vi "v4.11.vi"() -> ()   [LabVIEW 2018]
uses:
  <vilib>/DAQmx/read.llb/DAQmx Read (Analog 1D DBL NChan 1Samp).vi
  <extravilib>/ChannelInstances/High Speed Stream-c(a[.](c(dbl,dbl,dbl,dbl)),stamp,a[.](dbl),c(dbl,dbl,dbl,dbl,dbl,dbl,dbl))/_Read For Replicate.vi
  <extravilib>/ChannelInstances/High Speed Stream-c(a[.](c(dbl,dbl,dbl,dbl)),stamp,a[.](dbl),c(dbl,dbl,dbl,dbl,dbl,dbl,dbl))/Instantiate.vi
  <extravilib>/ChannelInstances/High Speed Stream-c(a[.](c(dbl,dbl,dbl,dbl)),stamp,a[.](dbl),c(dbl,dbl,dbl,dbl,dbl,dbl,dbl))/)Channel.vi
  <extravilib>/ChannelInstances/High Speed Stream-c(a[.](c(dbl,dbl,dbl,dbl)),stamp,a[.](dbl),c(dbl,dbl,dbl,dbl,dbl,dbl,dbl))/Abort Signal/Init Signal.vi
  <vilib>/Utility/file.llb/Write Delimited Spreadsheet (string).vi
  <vilib>/DAQmx/create/channels.llb/DAQmx Create Channel (AI-Temperature-Thermocouple).vi
  <vilib>/DAQmx/configure/timing.llb/DAQmx Timing (Sample Clock).vi
  <vilib>/DAQmx/miscellaneous.llb/DAQmx Fill In Error Info.vi
  <extravilib>/ChannelInstances/High Speed Stream-c(a[.](c(dbl,dbl,dbl,dbl)),stamp,a[.](dbl),c(dbl,dbl,dbl,dbl,dbl,dbl,dbl)).lvlib
  <resource>/objmgr/daqmx.rc
panel:
  out "Current Time":timestamp format="%<%X\n%x>T"
  out "Actual Sample Rate":dbl
  out "Rig Temperatures":T1
  out "Flowrate Data":T2(array[cluster])
  out "UI Timestamp":timestamp format="%<%X\n%x>T"
  out "DAQ Timestamp":timestamp format="%<%H:%M:%S>T"
  in  "file path (dialog if empty)":path
  out "Output\nStatus":T3(ring)
  in  "Start Recording?":bool
  in  "Stop Recording?":bool
  in  "Flowrate Control":dbl
  out "Status":T4(ring)
  in  "OK Button":bool
  in  "DAQ Properties":cluster{"Sample Rate [Hz]":dbl}={"Sample Rate [Hz]"=1.0} {"Sample Rate [Hz]" min=0.1 max=10000.0 step=0.1}
  # "Line Data"
  # "Rig Temperatures [ °C]"
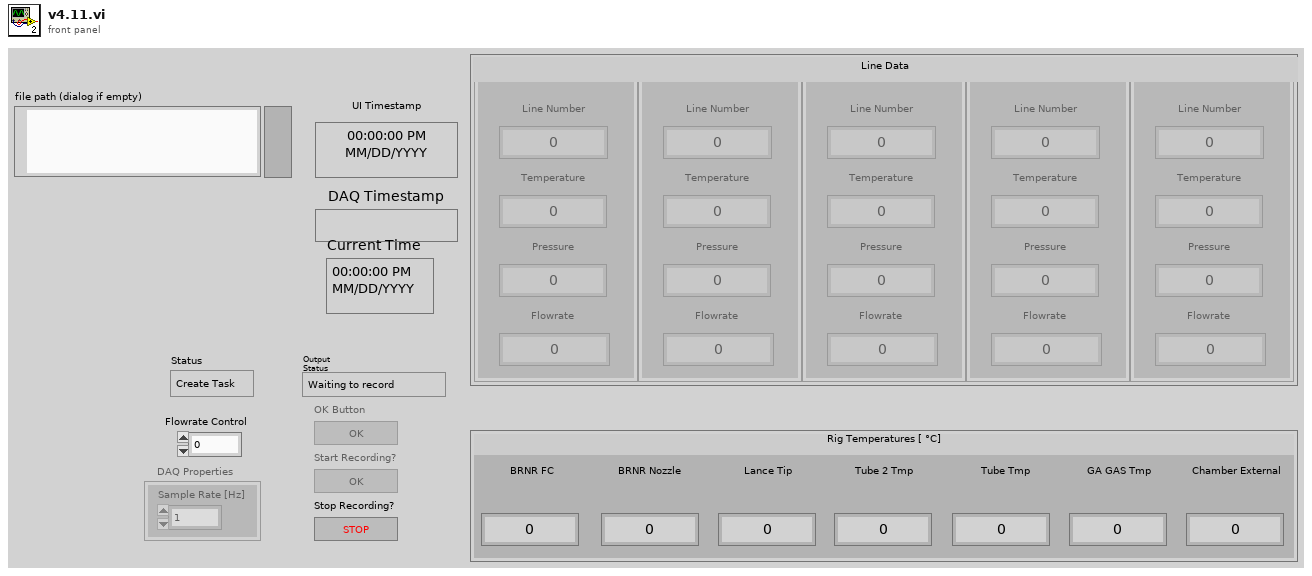
[diagram p1: front panel]
types:
  T1 = cluster{"BRNR FC":dbl, "BRNR Nozzle":dbl, "Lance Tip":dbl, "Tube 2 Tmp":dbl, "Tube Tmp":dbl, "GA GAS Tmp":dbl, "Chamber External":dbl}
  T2 = cluster{"Line Number":dbl, "Temperature":dbl, "Pressure":dbl, "Flowrate":dbl}[]
  T3 = enum16{"Waiting to record", "Creating Spreadsheet", "Recording", "Finished Recording"}
  T4 = enum16{"Create Task", "Change Settings", "Check Settings", "Read Data", "End Task"}
  T5 = enum8{"Enabled", "Disabled", "Disabled and Grayed Out"}
  T6 = cluster{"Flowrate Data":cluster{"Line Number":dbl, "Temperature":dbl, "Pressure":dbl, "Flowrate":dbl}[], "Current Time":timestamp, "DAQmx Data":dbl[], "Rig Temperatures":cluster{"BRNR FC":dbl, "BRNR Nozzle":dbl, "Lance Tip":dbl, "Tube 2 Tmp":dbl, "Tube Tmp":dbl, "GA GAS Tmp":dbl, "Chamber External Temp":dbl}}
  T7 = cluster{"BRNR FC":dbl, "BRNR Nozzle":dbl, "Lance Tip":dbl, "Tube 2 Tmp":dbl, "Tube Tmp":dbl, "GA GAS Tmp":dbl, "Chamber External Temp":dbl}
  T8 = typedef "High Speed Stream-c(a[.](c(dbl,dbl,dbl,dbl)),stamp,a[.](dbl),c(dbl,dbl,dbl,dbl,dbl,dbl,dbl)).lvlib/)Channel.ctl" = refnum<queue>
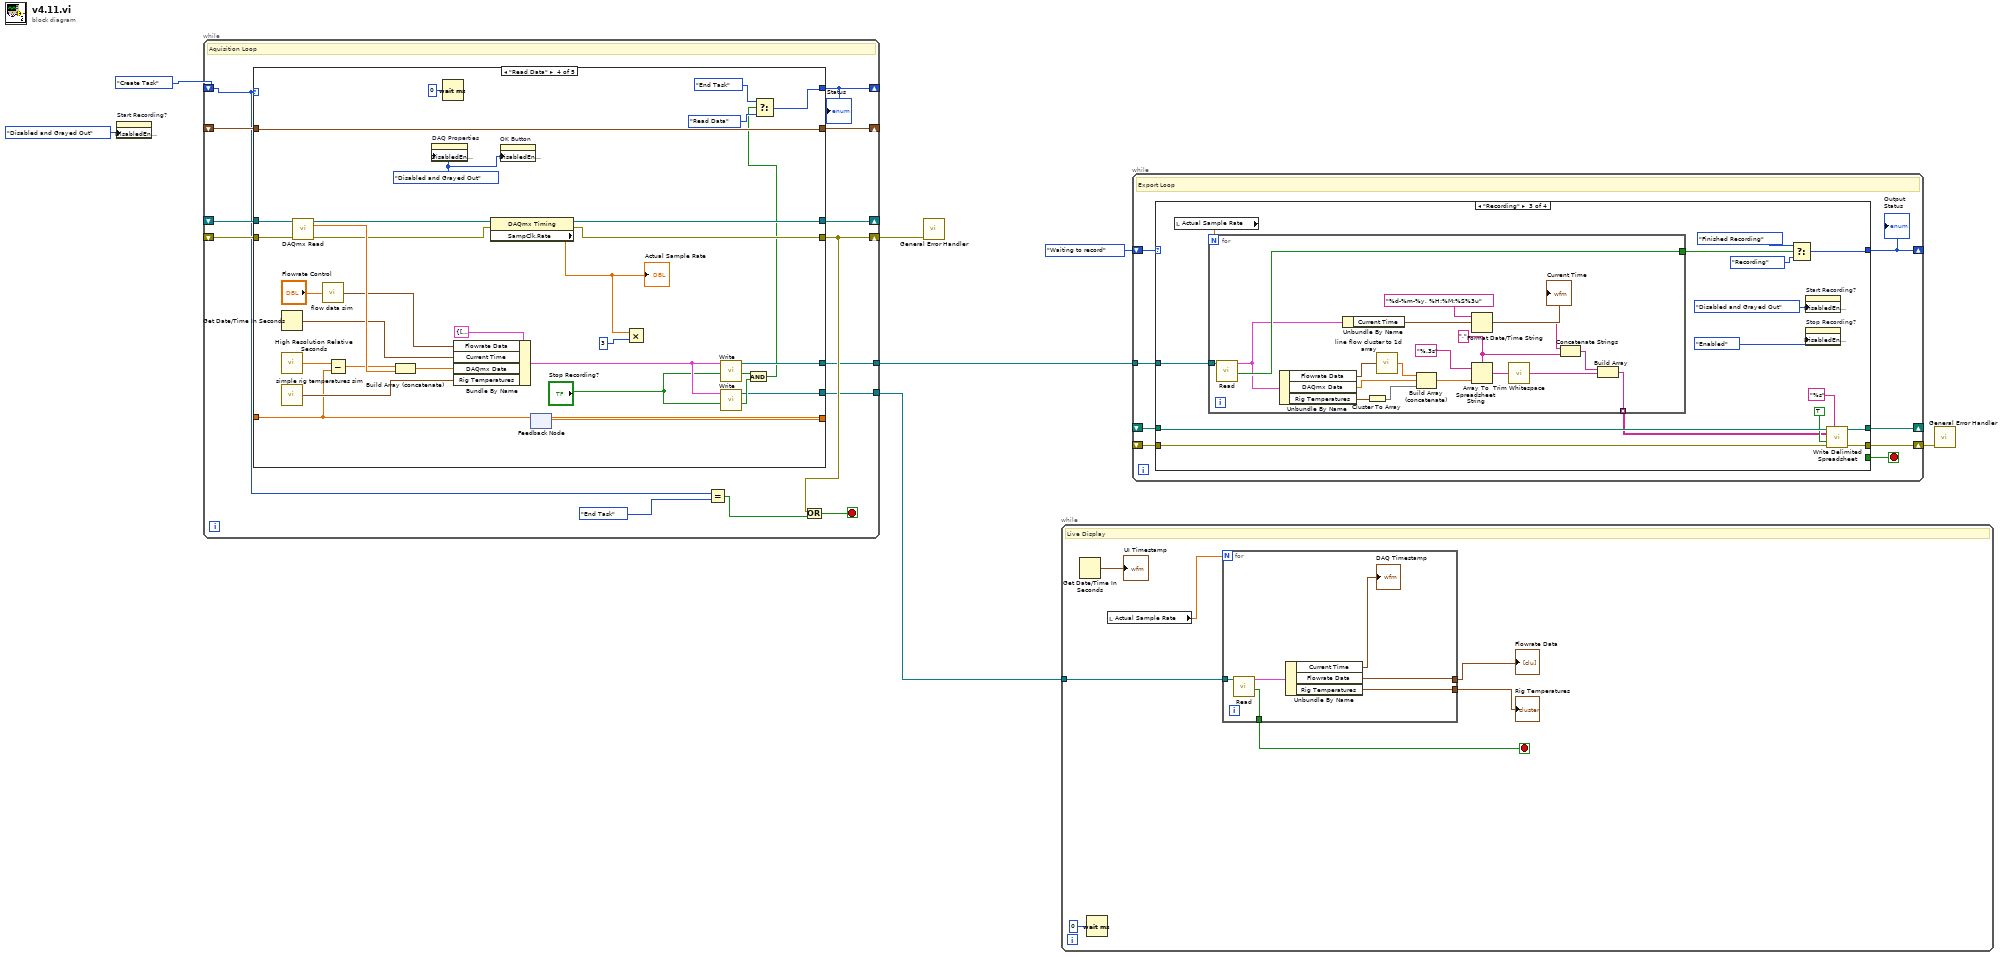
[diagram p0: block diagram]
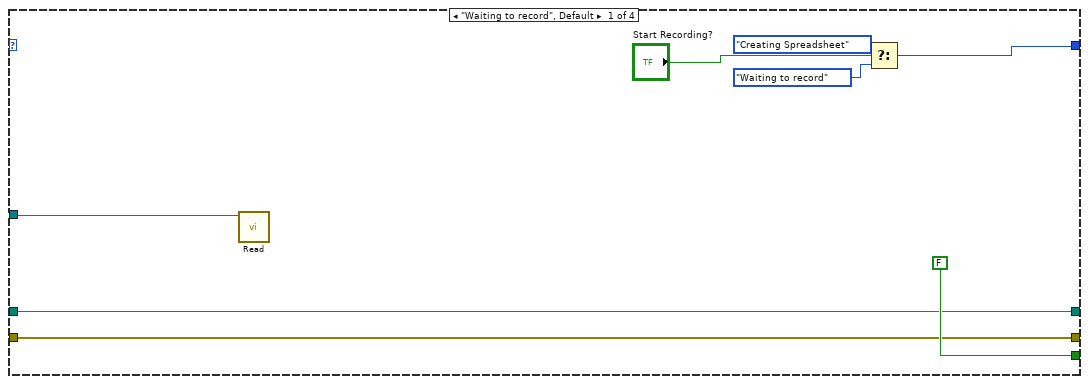
[diagram p2: hidden frame]
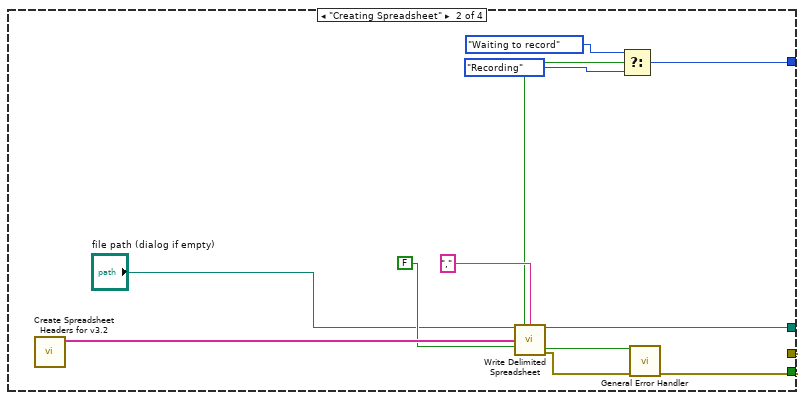
[diagram p3: hidden frame]
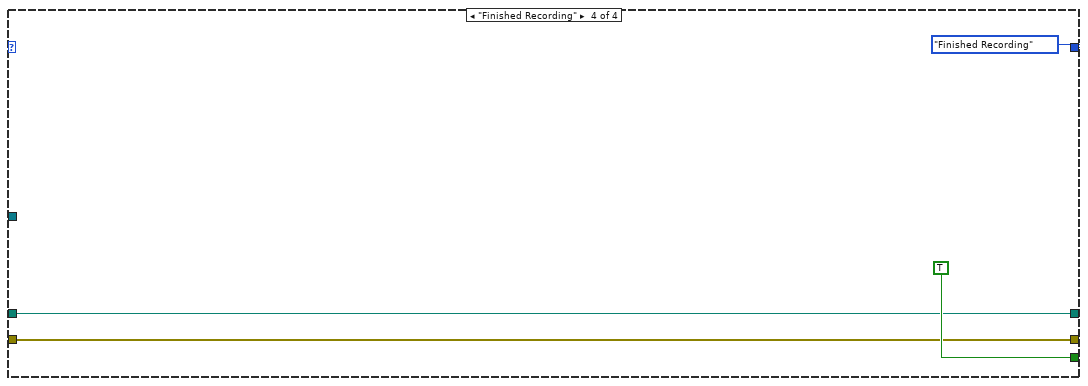
[diagram p4: hidden frame]
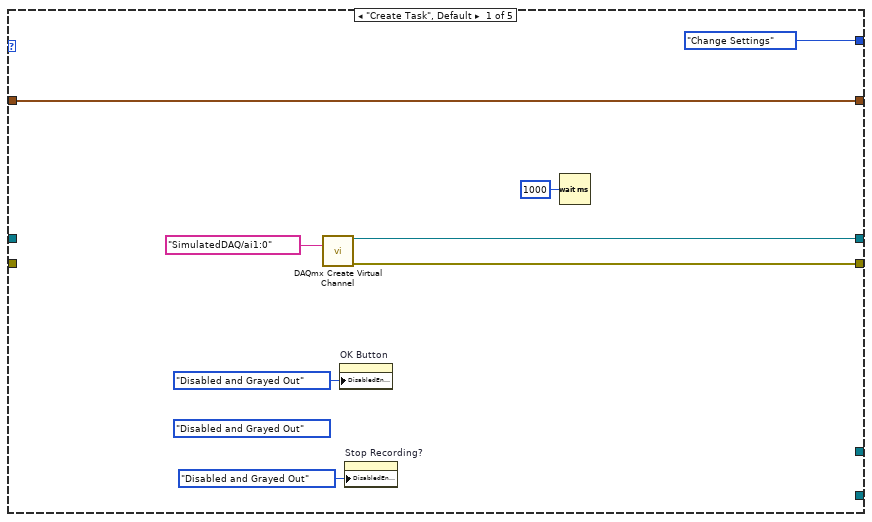
[diagram p5: hidden frame]
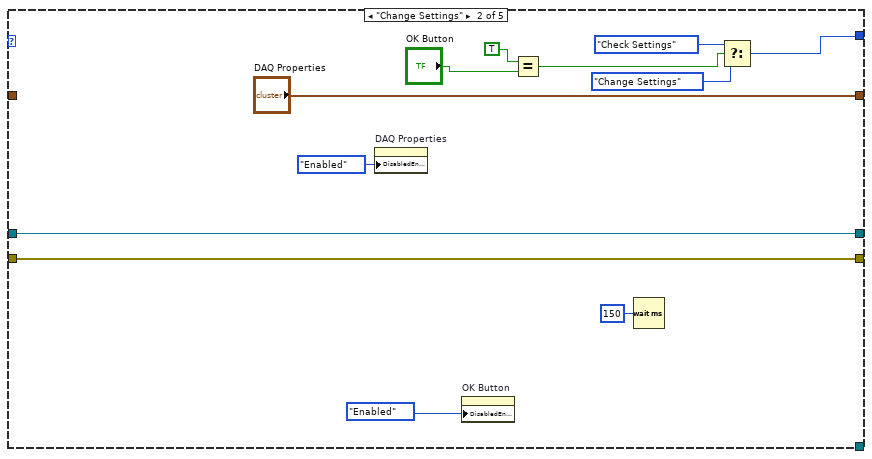
[diagram p6: hidden frame]
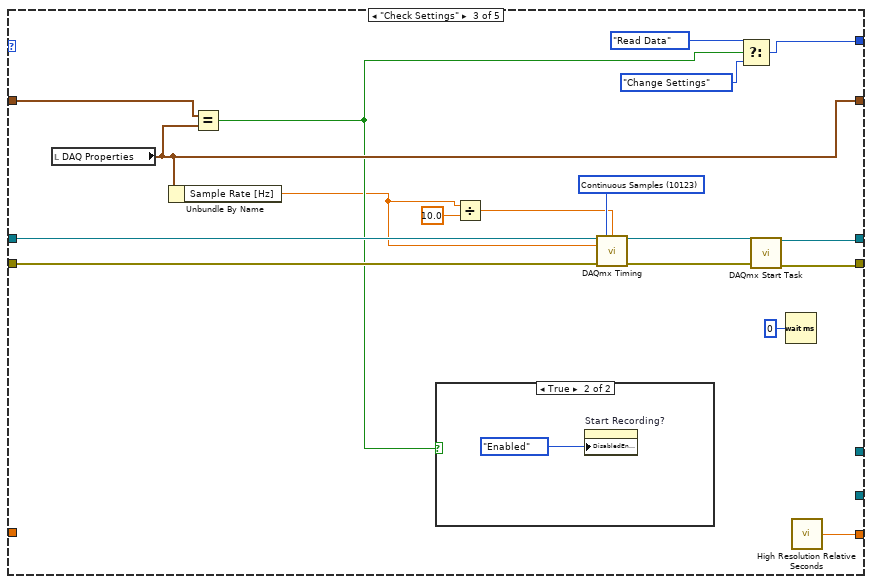
[diagram p7: hidden frame]
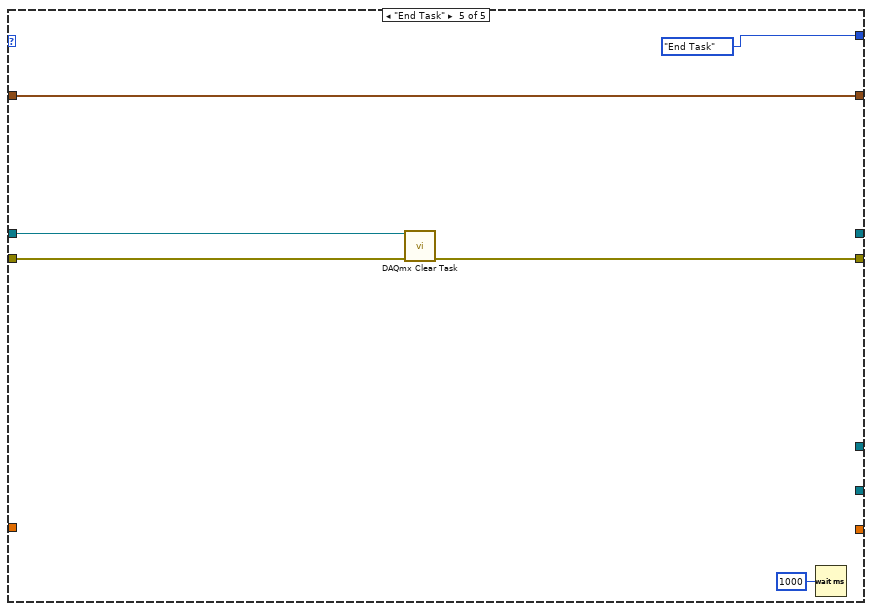
[diagram p9: hidden frame]
diagram:
  n1 = property on="Start Recording?" class="Bool"("DisabledEnum"=T5."Disabled and Grayed Out" ("Disabled")) -> ()  [unwired: 2 in, 2 out]
  n2 = while {
    shift-right: [w17] -> _
    shift-left: T4."Create Task" -> [w13]
    shift-right: [w22] -> _
    shift-left: _ -> [w20]
    shift-right: [w16] -> w3
    shift-left: _ -> [w19]
    shift-right: [w21] -> _
    shift-left: _ -> [w18]
    tunnel: [w11] -> w5
    tunnel: [w10] -> w1
    stop <- w12 stop-if-true
    # "Aquisition Loop"
    n3 = feedback #1() -> (w8:dbl)  [unwired: 1 in]
    n4 = case shown="\"Read Data\"" w13 {
      tunnel: [w30 w42 w50 w72 _] -> w22
      tunnel: [w29 w41 w49 w73 w98] -> w16
      tunnel: [T4."Change Settings" w35 w56 w88 T4."End Task"] -> w17
      tunnel: [w26 "DAQ Properties" w53 w90 w97] -> w21
      tunnel: w20 -> [_ w42 w55 w92 w95]
      tunnel: w19 -> [_ w41 w54 w91 w94]
      tunnel: w18 -> [w26 _ w60 w90 w97]
      tunnel: [_ _ _ w79 _] -> w11
      tunnel: [_ _ _ w70 _] -> w10
      tunnel: [_ _ w43 w65 _] -> w9
      tunnel: w8 -> [_ _ _ w65 _]
      frame "Create Task", Default {
        (unwired) T5."Disabled and Grayed Out" ("Disabled")
        n5 = call-poly <vilib>:"DAQmx Create Virtual Channel.vi"("physical channels"=tag "SimulatedDAQ/ai1:0") -> ("task out"=w30:refnum<k21>, "error out"=w29:errorcluster)  [unwired: 13 in]
        n6 = property on="OK Button" class="Bool"("DisabledEnum"=T5."Disabled and Grayed Out" ("Disabled")) -> ()  [unwired: 2 in, 2 out]
        n7 = property on="Stop Recording?" class="Bool"("DisabledEnum"=T5."Disabled and Grayed Out" ("Disabled")) -> ()  [unwired: 2 in, 2 out]
        n8 = Wait (ms)(milliseconds to wait=u32 1000) -> ()  [unwired: 1 out]
      }
      frame "Change Settings" {
        n9 = property on="DAQ Properties" class="Clust (strict)"("DisabledEnum"=T5."Enabled" ("Disabled")) -> ()  [unwired: 2 in, 2 out]
        n10 = property on="OK Button" class="Bool"("DisabledEnum"=T5."Enabled" ("Disabled")) -> ()  [unwired: 2 in, 2 out]
        n11 = Equal?(x=TRUE, y="OK Button") -> (x = y?=w37:bool)
        n12 = Wait (ms)(milliseconds to wait=u32 150) -> ()  [unwired: 1 out]
        n13 = Select(t=T4."Check Settings", s=w37, f=T4."Change Settings") -> (s? t:f=w35:T4)
      }
      frame "Check Settings" {
        w48 = 10123 items=["Finite Samples"=10178, "Continuous Samples"=10123, "Hardware Timed Single Point"=12522] ("sample mode")
        n14 = local read "DAQ Properties"() -> (w53:cluster{"Sample Rate [Hz]":dbl})
        n15 = Unbundle By Name(w53) -> ("Sample Rate [Hz]"=w45:dbl)
        n16 = Equal?(x=w60, y=w53) -> (x = y?=w47:bool)
        n17 = case shown="True" w47 {
          frame False {
          }
          frame True {
            n18 = property on="Start Recording?" class="Bool"("DisabledEnum"=T5."Enabled" ("Disabled")) -> ()  [unwired: 2 in, 2 out]
          }
        }
        n19 = Divide(x=w45, y=10.0) -> (x/y=w44:dbl)
        n20 = call-poly <vilib>:"DAQmx Timing.vi"("task/channels in"=w55, "sample mode"=w48, "samples per channel"=w44, "rate"=w45, "error in"=w54) -> ("task out"=w52:refnum<k21>, "error out"=w51:errorcluster)  [unwired: 9 in]
        n21 = Select(t=T4."Read Data", s=w47, f=T4."Change Settings") -> (s? t:f=w56:T4)
        n22 = call <vilib>:"DAQmx Start Task.vi"("task/channels in"=w52, "error in"=w51) -> ("task out"=w50:refnum<k21>, "error out"=w49:errorcluster)  [unwired: 12 in]
        n23 = Wait (ms)(milliseconds to wait=u32 0) -> ()  [unwired: 1 out]
        n24 = call <vilib>:"High Resolution Relative Seconds.vi"() -> ("relative seconds"=w43:dbl)
      }
      frame "Read Data" {
        w78 = T5."Disabled and Grayed Out" ("Disabled")
        n25 = Get Date/Time In Seconds() -> (seconds since 1Jan1904=w82:timestamp)
        n26 = call <vilib>:"High Resolution Relative Seconds.vi"() -> ("relative seconds"=w69:dbl)
        n27 = call "simple rig temperatures sim.vi"() -> ("Rig Temperatures"=w80:T7)
        n28 = call-poly <vilib>:"DAQmx Read.vi"("task/channels in"=w92, "error in"=w91) -> ("task out"=w74:refnum<k21>, "data"=w85:dbl[], "error out"=w71:errorcluster)  [unwired: 11 in]
        n29 = call "flow data sim.vi"("Boondoggle Input"="Flowrate Control") -> ("Flowrate Data"=w81:T2)
        n30 = Subtract(x=w69, y=w65) -> (x-y=w66:dbl)
        n31 = Build Array (concatenate)(w66, w85) -> (w67:dbl[])
        n32 = property on="DAQ Properties" class="Clust (strict)"("DisabledEnum"=w78) -> ()  [unwired: 2 in, 2 out]
        n33 = Wait (ms)(milliseconds to wait=u32 0) -> ()  [unwired: 1 out]
        n34 = Bundle By Name(cluster=T6 {"Flowrate Data"=[{"Line Number"=1.0, "Temperature"=17.480721541683437, "Pressure"=24.0, "Flowrate"=0.0}, {"Line Number"=2.0, "Temperature"=21.850901927104296, "Pressure"=30.0, "Flowrate"=0.0}, {"Line Number"=3.0, "Temperature"=26.221082312525155, "Pressure"=36.0, "Flowrate"=0.0}, {"Line Number"=4.0, "Temperature"=30.591262697946018, "Pressure"=42.00000000000001, "Flowrate"=0.0}, {"Line Number"=5.0, "Temperature"=34.96144308336687, "Pressure"=48.0, "Flowrate"=0.0}], "Current Time"=timestamp(0 s since 1904-01-01), "DAQmx Data"=[], "Rig Temperatures"={"BRNR FC"=0.0, "BRNR Nozzle"=0.0, "Lance Tip"=0.0, "Tube 2 Tmp"=0.0, "Tube Tmp"=0.0, "GA GAS Tmp"=0.0, "Chamber External Temp"=0.0}}, "Flowrate Data"=w81, "Current Time"=w82, "DAQmx Data"=w67, "Rig Temperatures"=w80) -> (w77:T6)
        n35 = property class="DAQmx Timing"(reference=w74, error in=w71) -> (reference out=w72:refnum<k21>, error out=w73:errorcluster, "SampClk.Rate"=w64:dbl)
        "Actual Sample Rate" <- w64
        n36 = property on="OK Button" class="Bool"("DisabledEnum"=w78) -> ()  [unwired: 2 in, 2 out]
        n37 = Multiply(x=w64, y=3) -> ()  [unwired: 1 out]
        n38 = call <extravilib>:"Write.vi"("last element? (F)"="Stop Recording?", "element"=w77) -> ("done?"=w76:bool, "channel"=w79:T8)  [unwired: 7 in, 1 out]
        n39 = call <extravilib>:"Write.vi"("last element? (F)"="Stop Recording?", "element"=w77) -> ("done?"=w75:bool, "channel"=w70:T8)  [unwired: 7 in, 1 out]
        n40 = And(x=w76, y=w75) -> (x .and. y?=w68:bool)
        n41 = Select(t=T4."End Task", s=w68, f=T4."Read Data") -> (s? t:f=w88:T4)
      }
      frame "End Task" {
        n42 = call <vilib>:"DAQmx Clear Task.vi"("task in"=w95, "error in"=w94) -> ("error out"=w98:errorcluster)  [unwired: 13 in]
        n43 = Wait (ms)(milliseconds to wait=u32 1000) -> ()  [unwired: 1 out]
      }
    }
    "Status" <- w17
    n44 = feedback-in #1(w9) -> ()
    n45 = Equal?(x=w13, y=T4."End Task") -> (x = y?=w14:bool)
    n46 = Or(x=w16, y=w14) -> (x .or. y?=w12:bool)
  }
  n47 = call <vilib>:"General Error Handler.vi"("error in (no error)"=w3) -> ()  [unwired: 10 in, 5 out]
  n48 = while {
    tunnel: w1 -> [w102]
    stop <- w105 stop-if-true
    # "Live Display"
    n49 = Get Date/Time In Seconds() -> (seconds since 1Jan1904=→"UI Timestamp":timestamp)
    n50 = Wait (ms)(milliseconds to wait=u32 0) -> ()  [unwired: 1 out]
    n51 = local read "Actual Sample Rate"() -> (w101:dbl)
    n52 = for {
      N: w101 -> [_]
      tunnel: [w111] -> w105
      tunnel: w102 -> [w108]
      tunnel: [w107] -> w99
      tunnel: [w106] -> w100
      n53 = call <extravilib>:"Read.vi"("channel"=w108) -> ("done?"=w111:bool, "element"=w110:T6)  [unwired: 6 in, 3 out]
      n54 = Unbundle By Name(w110) -> ("Current Time"=→"DAQ Timestamp":timestamp, "Flowrate Data"=w107:T2, "Rig Temperatures"=w106:T7)
    }
    "Flowrate Data" <- w99
    "Rig Temperatures" <- w100
  }
  n55 = while {
    shift-right: [w119] -> _
    shift-left: T3."Waiting to record" -> [w118]
    tunnel: w5 -> [w116]
    shift-right: [w114] -> _
    shift-left: _ -> [w115]
    shift-right: [w113] -> w4
    shift-left: _ -> [w112]
    stop <- w117 stop-if-true
    # "Export Loop"
    n56 = case shown="\"Recording\"" w118 {
      tunnel: [w124 w130 w152 T3."Finished Recording"] -> w119
      tunnel: [FALSE _ _ TRUE] -> w117
      tunnel: w116 -> [w120 _ w149 _]
      tunnel: w115 -> [w122 _ w146 w173]
      tunnel: [w122 w138 w147 w173] -> w114
      tunnel: [w121 w132 w142 w172] -> w113
      tunnel: w112 -> [w121 _ w145 w172]
      frame "Waiting to record", Default {
        n57 = call <extravilib>:"Read.vi"("channel"=w120) -> ()  [unwired: 6 in, 5 out]
        n58 = Select(t=T3."Creating Spreadsheet", s="Start Recording?", f=T3."Waiting to record") -> (s? t:f=w124:T3)
      }
      frame "Creating Spreadsheet" {
        n59 = call "Create Spreadsheet Headers for v3.2.vi"() -> ("Array"=w137:string[])  [unwired: 11 in]
        n60 = call-poly <vilib>:"Write Delimited Spreadsheet.vi"("file path (dialog if empty)"="file path (dialog if empty)", "1D data"=w137, "append to file? (new file:F)"=FALSE, "delimiter (\\t)"="," ("delimiter (\\t)")) -> ("new file path (Not A Path if cancelled)"=w138:path, "error out"=w133:errorcluster)  [unwired: 10 in]
        n61 = call <vilib>:"General Error Handler.vi"("error in (no error)"=w133) -> ("error?"=w131:bool, "error out"=w132:errorcluster)  [unwired: 10 in, 3 out]
        n62 = Select(t=T3."Waiting to record", s=w131, f=T3."Recording") -> (s? t:f=w130:T3)
      }
      frame "Recording" {
        n63 = local read "Actual Sample Rate"() -> (w139:dbl)
        n64 = for {
          N: w139 -> [_]
          tunnel: w149 -> [w170]
          tunnel: [w169] -> w148
          tunnel: [w154] -> w140 mode=indexing
          w159 = "," ("delimiter (Tab)")
          n65 = call <extravilib>:"Read.vi"("channel"=w170) -> ("done?"=w169:bool, "element"=w167:T6)  [unwired: 6 in, 3 out]
          n66 = Unbundle By Name(w167) -> ("Flowrate Data"=w168:T2, "DAQmx Data"=w165:dbl[], "Rig Temperatures"=w171:T7)
          n67 = Unbundle By Name(w167) -> ("Current Time"=w160:timestamp)
          "Current Time" <- w160
          n68 = Cluster To Array(cluster=w171) -> (array=w166:dbl[])
          n69 = call "line flow cluster to 1d array.vi"("Flowrate Data"=w168) -> ("Array"=w164:dbl[])
          n70 = Build Array (concatenate)(w164, w165, w166) -> (w157:dbl[])
          n71 = Format Date/Time String(time format string (%c)="%d-%m-%y, %H:%M:%S%3u", seconds (now)=w160) -> (date/time string=w158:string)  [unwired: 1 in]
          n72 = Array To Spreadsheet String(delimiter (Tab)=w159, array=w157, 3:"%.3s" ("format string")) -> (spreadsheet string=w163:string)
          n73 = call <vilib>:"Trim Whitespace.vi"("string"=w163) -> ("trimmed string"=w155:string)  [unwired: 1 in]
          n74 = Concatenate Strings(w158, w159) -> (w156:string)
          n75 = Build Array(w156, w155) -> (w154:string[])
        }
        n76 = Select(t=T3."Finished Recording", s=w148, f=T3."Recording") -> (s? t:f=w152:T3)
        n77 = property on="Start Recording?" class="Bool"("DisabledEnum"=T5."Disabled and Grayed Out" ("Disabled")) -> ()  [unwired: 2 in, 2 out]
        n78 = property on="Stop Recording?" class="Bool"("DisabledEnum"=T5."Enabled" ("Disabled")) -> ()  [unwired: 2 in, 2 out]
        n79 = call-poly <vilib>:"Write Delimited Spreadsheet.vi"("file path (dialog if empty)"=w146, "format (%s)"="%s", "2D data"=w140, "append to file? (new file:F)"=TRUE, "error in (no error)"=w145) -> ("new file path (Not A Path if cancelled)"=w147:path, "error out"=w142:errorcluster)  [unwired: 9 in]
      }
      frame "Finished Recording" {
      }
    }
    "Output\nStatus" <- w119
  }
  n80 = call <vilib>:"General Error Handler.vi"("error in (no error)"=w4) -> ()  [unwired: 10 in, 5 out]
